vi "TCP Client.vi"() -> ()   [LabVIEW 2016, in "流量计集成.lvlib" / "LS-H600流量计.lvlib"]
panel:
  in  "远程端口或服务名称":u16=5007
  in  "地址":string="localhost"
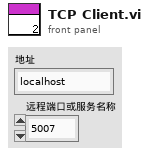
[diagram p1: front panel]
types:
  T1 = enum16{"open TCP", "Read TCP", "Decode", "Close TCP"}
  T2 = enum16{"Standard", "Buffered", "CRLF", "Immediate"}
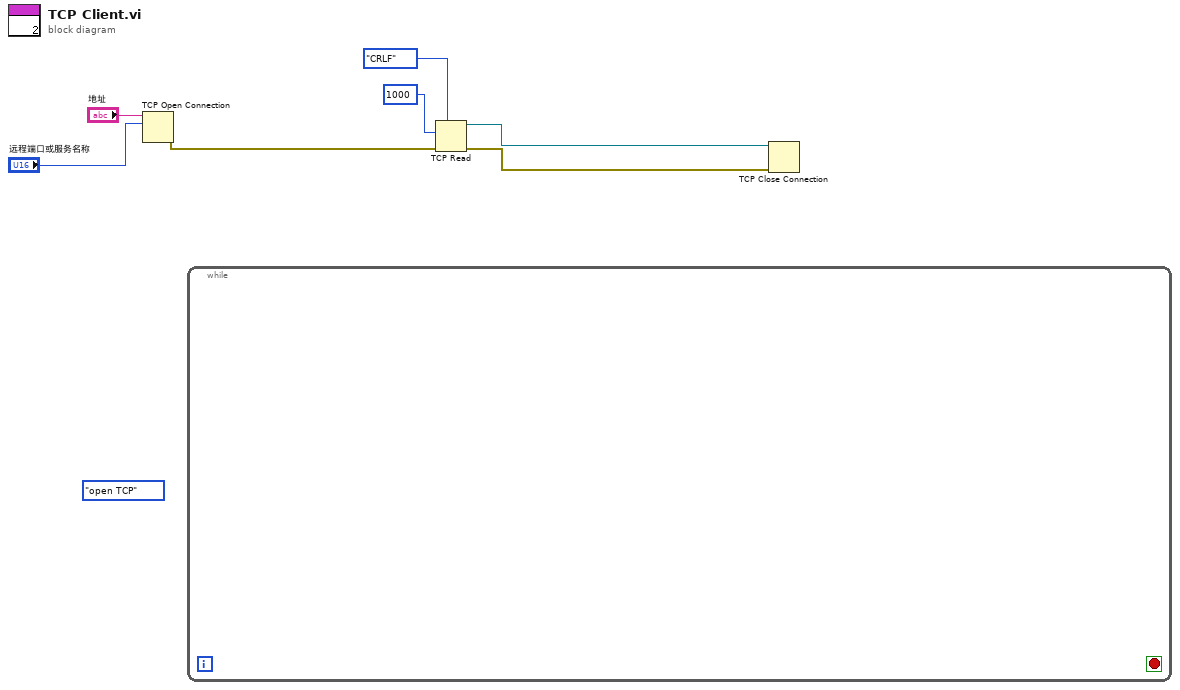
[diagram p0: block diagram]
diagram:
  (unwired) T1."open TCP" ("枚举")
  n1 = TCP Open Connection(address="地址", remote port or service name="远程端口或服务名称") -> (error out=w5:errorcluster)  [unwired: 3 in, 1 out]
  n2 = while {
    stop <- _ stop-if-true
  }
  n3 = TCP Read(bytes to read=1000 ("读取的字节"), error in (no error)=w5, 7:T2."CRLF" ("模式（标准）")) -> (connection ID out=w2:refnum<k5>, error out=w1:errorcluster)  [unwired: 2 in, 1 out]
  n4 = TCP Close Connection(connection ID=w2, error in (no error)=w1) -> ()  [unwired: 1 in, 2 out]
